vi "VCU MODEL CAN0.vi"() -> ()   [LabVIEW 2015]
uses:
  <vilib>/FPGAPlugInAG/cRIO-9063/niLvFpga_Open_cRIO-9063.vi
  <vilib>/rvi/interface/common/dynamic/niFpgaDynamicAddResources.vi
  <vilib>/Utility/error.llb/Error Cluster From Error Code.vi
  <vilib>/rvi/errors/niLvFpgaAdjustHostInterfaceError.vi
  <vilib>/FPGAPlugInAG/Dynamic/niLvFpga_Close_Dynamic.vi
  <vilib>/rvi/interface/nirviOpenFPGA/nirviOpenFPGA.xnode
  FPGA Bitfiles/VCU-VEHICLEMODEL_FPGATarget_CANBasic(FPGA)_WVt1gIpoBPw.lvbitx
  Basic (FPGA) CAN Engine .vi
  <vilib>/rvi/interface/nirviReadWriteControl/nirviReadWriteControl.xnode
  <vilib>/rvi/interface/nirviCloseFPGA/nirviCloseFPGA.xnode
  <vilib>/rvi/interface/Simulation/niFpgaSimulationCallBeginRW.vi
  NiFpgaLv.dll
panel:
  in  "Route_leg":u16
  in  "Start":bool
  out "P":cluster{sgl, sgl}(graph)
  out "V":cluster{"Vx_PV":sgl, "Vy_PV":sgl}(graph)
  out "Loop time":sgl
  out "Old Timestamp":u64
  out "Timestamp":u64
  out "Delta_Px":sgl
  out "Delta_Vx":sgl
  out "Delta_Py":sgl
  out "Delta_Vy":sgl
  out "F_C (magnitude)":sgl
  out "Theta_C (direction)":sgl
  out "Vx_SP":sgl
  out "x_MV (SGL)":sgl
  out "x_MV+ (plus m_epsilon)":sgl
  out "y_MV (SGL)":sgl
  out "Vy_SP":sgl
  out "Inverse Tangent (SGL)":sgl
  in  "Px_SP":sgl
  in  "Py_SP":sgl
  out "Vy_PV":sgl
  out "Px_PV":sgl
  out "Py_PV":sgl
  out "Vx_PV":sgl
  out "No# Frames Received":i32
  out "No# Frames Sent":i32
  out "error out":errorcluster
  # "Output"
  # "Set Point"
  # "Sensor Values"
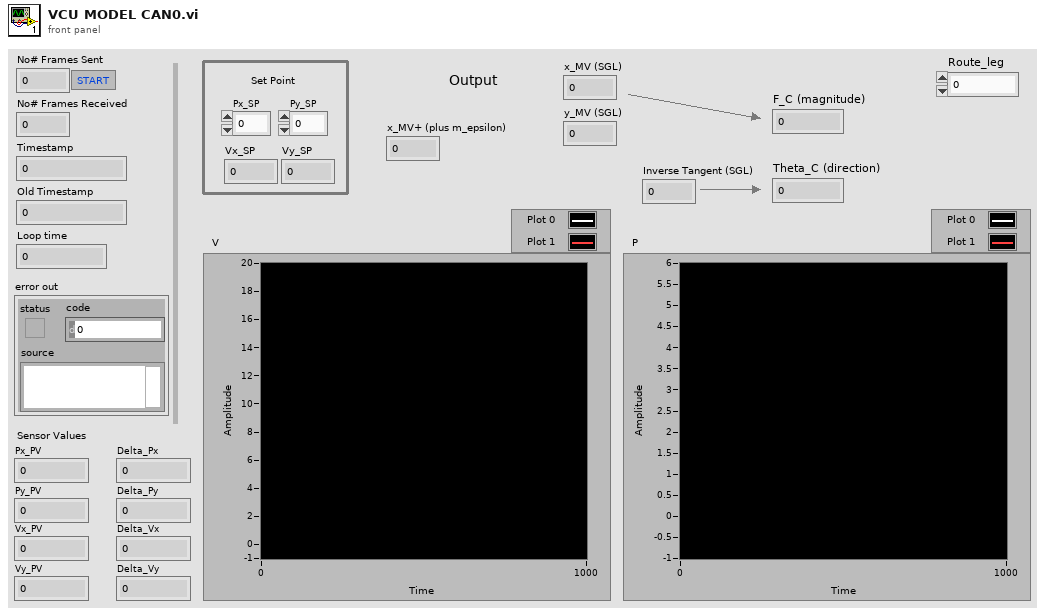
[diagram p1: front panel]
types:
  T1 = enum8{"Data Frame", "Remote Frame", "(reserved)", "(reserved) ", "(reserved)  ", "(reserved)   ", "Bus Error", "Transceiver Fault"}
  T2 = cluster{"timestamp high":u32, "timestamp low":u32, "identifier":u32, "type":enum8{"Data Frame", "Remote Frame", "(reserved)", "(reserved) ", "(reserved)  ", "(reserved)   ", "Bus Error", "Transceiver Fault"}, "info A":u8, "info B":u8, "data length":u8, "data":u8[]}
  T3 = cluster{u32, u32, u32, "type":enum8{"Data Frame", "Remote Frame", "(reserved)", "(reserved) ", "(reserved)  ", "(reserved)   ", "Bus Error", "Transceiver Fault"}, u8, u8, u8, u8[]}
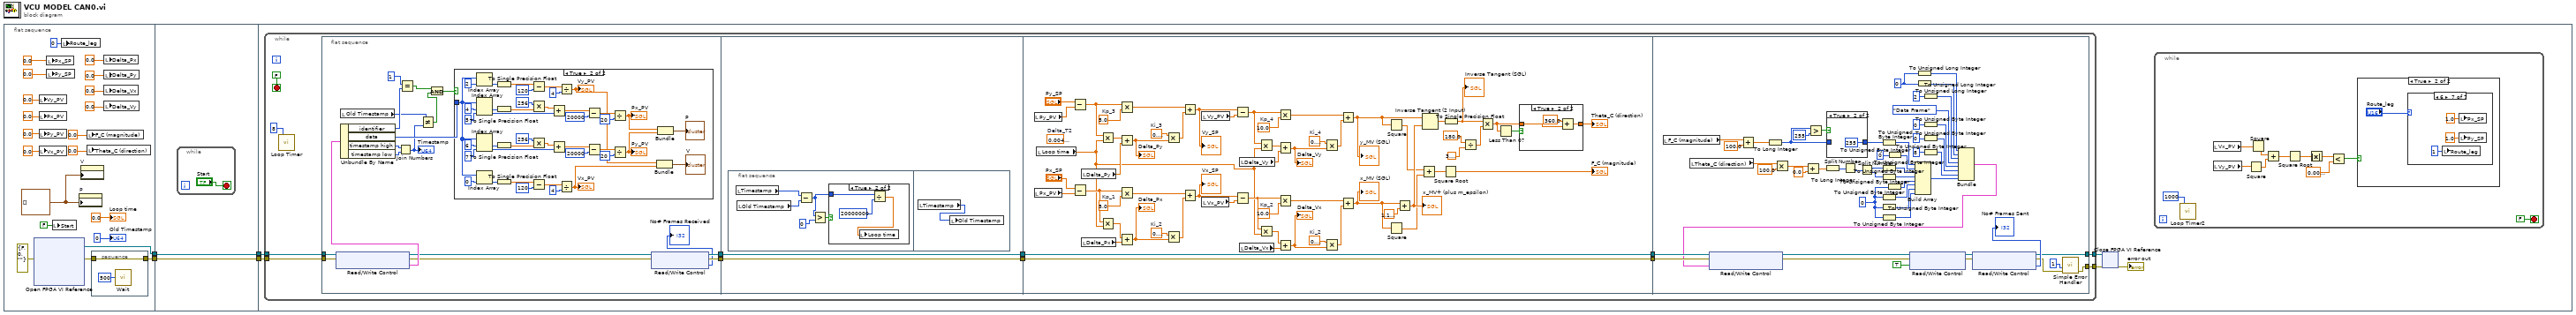
[diagram p0: block diagram]
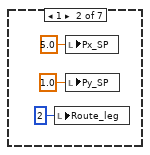
[diagram p4: hidden frame]
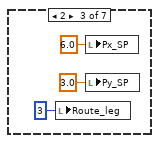
[diagram p5: hidden frame]
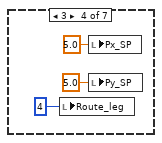
[diagram p6: hidden frame]
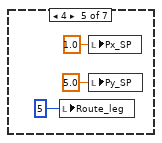
[diagram p7: hidden frame]
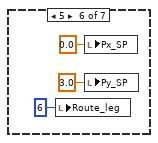
[diagram p8: hidden frame]
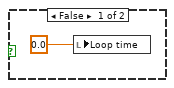
[diagram p10: hidden frame]
diagram:
  n1 = flat-sequence {
    tunnel: [w11] -> w4
    tunnel: [w10] -> w2
    tunnel: w4 -> [w29]
    tunnel: [w29] -> w3
    tunnel: w2 -> [w28]
    tunnel: [w28] -> w1
    tunnel: w3 -> [w32]
    tunnel: w1 -> [w31]
    frame #0 {
      w7 = cluster{"Px_PV":sgl, "Py_PV":sgl}[] [] ("History Data")
      n2 = xnode "Open FPGA VI Reference"("error in"=errorcluster {"status"=FALSE, "code"=0, "source"=""}) -> ("FPGA VI Reference Out"=w10:refnum<k20>, "error out"=w12:errorcluster)  [unwired: 1 in]
      n3 = local write "Vy_PV"(sgl 0.0 ("Vx_C")) -> ()
      n4 = local write "Px_PV"(sgl 0.0 ("Vy_C")) -> ()
      n5 = local write "Py_PV"(sgl 0.0 ("Px_C")) -> ()
      n6 = local write "Vx_PV"(sgl 0.0 ("Py_C")) -> ()
      n7 = local write "Px_SP"(sgl 0.0 ("Vx_C")) -> ()
      n8 = local write "Py_SP"(sgl 0.0 ("Vx_C")) -> ()
      n9 = local write "Start"(FALSE ("Start")) -> ()
      n10 = local write "Route_leg"(u16 0 ("Route_leg")) -> ()
      n11 = property on="P" class="WFChart (strict)"("History Data"=w7) -> ()  [unwired: 2 in, 2 out]
      n12 = property on="V" class="WFChart (strict)"("History Data"=w7) -> ()  [unwired: 2 in, 2 out]
      n13 = local write "F_C (magnitude)"(sgl 0.0 ("F_C")) -> ()
      n14 = local write "Theta_C (direction)"(sgl 0.0 ("Theta_C")) -> ()
      n15 = stacked-sequence {
        tunnel: w12 -> [w27]
        tunnel: [w27] -> w11
        frame #0 {
          n16 = call "Wait"("Count(mSec)"=u32 500) -> ()  [unwired: 1 out]
        }
      }
      n17 = local write "Delta_Px"(sgl 0.0 ("Delta_Px")) -> ()
      n18 = local write "Delta_Py"(sgl 0.0 ("Delta_Py")) -> ()
      n19 = local write "Delta_Vx"(sgl 0.0 ("Delta_Vx")) -> ()
      n20 = local write "Delta_Vy"(sgl 0.0) -> ()
      "Loop time" <- sgl 0.0 ("Loop time")
      "Old Timestamp" <- u64 0 ("Old Timestamp")
    }
    frame #1 {
      n21 = while {
        stop <- "Start" stop-if-true
      }
    }
    frame #2 {
      n22 = while {
        tunnel: [w76] -> w34
        tunnel: [w75] -> w33
        tunnel: w31 -> [w67]
        tunnel: w32 -> [w66]
        stop <- FALSE stop-if-true
        n23 = call "Loop Timer"("Count(mSec)"=u32 8) -> ()  [unwired: 1 out]
        n24 = flat-sequence {
          tunnel: [w91] -> w74
          tunnel: [w90] -> w72
          tunnel: w67 -> [w84]
          tunnel: w66 -> [w83]
          tunnel: w74 -> [w138]
          tunnel: [w138] -> w73
          tunnel: w72 -> [w137]
          tunnel: [w137] -> w71
          tunnel: w73 -> [w157]
          tunnel: w71 -> [w156]
          tunnel: [w157] -> w69
          tunnel: [w156] -> w68
          tunnel: [w214] -> w76
          tunnel: [w216] -> w75
          tunnel: w69 -> [w218]
          tunnel: w68 -> [w213]
          frame #0 {
            n25 = xnode "Read/Write Control"("FPGA VI Reference In"=w84, "error in"=w83) -> ("FPGA VI Reference Out"=w89:refnum<k20>, "error out"=w88:errorcluster, "CAN0 - Received Frame"=w94:T2)
            n26 = Unbundle By Name(w94) -> ("identifier"=w92:u32, "data"=w93:u8[], "timestamp high"=w86:u32, "timestamp low"=w85:u32)
            n27 = local read "Old Timestamp"() -> (w82:u64)
            n28 = Join Numbers(hi=w86, lo=w85) -> ((hi.lo)=w81:u64)
            "Timestamp" <- w81
            n29 = Equal?(x=u32 1, y=w92) -> (x = y?=w78:bool)
            n30 = Not Equal?(x=w82, y=w81) -> (x != y?=w79:bool)
            n31 = And(x=w78, y=w79) -> (x .and. y?=w80:bool)
            n32 = case shown="True" w80 {
              tunnel: w93 -> [_ w102]
              frame False {
              }
              frame True {
                n33 = Index Array(array=w102, index=2 ("索引")) -> (element=w110:u8)
                n34 = Index Array(array=w102, index #1=4 ("索引"), index #2=5 ("索引")) -> (element #1=w108:u8, element #2=w103:u8)
                n35 = Index Array(array=w102, index #1=6 ("索引"), index #2=7 ("索引")) -> (element #1=w106:u8, element #2=w122:u8)
                n36 = Index Array(array=w102, index=0 ("索引")) -> (element=w111:u8)
                n37 = To Single Precision Float(number=w110) -> (single precision float=w109:sgl)
                n38 = To Single Precision Float(number=w108) -> (single precision float=w107:sgl)
                n39 = To Single Precision Float(number=w106) -> (single precision float=w105:sgl)
                n40 = To Single Precision Float(number=w111) -> (single precision float=w112:sgl)
                n41 = Subtract(x=w109, y=u32 120) -> (x-y=w115:sgl)
                n42 = Multiply(x=u32 256 ("y"), y=w107) -> (x*y=w130:sgl)
                n43 = Multiply(x=u32 256 ("y"), y=w105) -> (x*y=w123:sgl)
                n44 = Subtract(x=w112, y=u32 120) -> (x-y=w135:sgl)
                n45 = Add(x=w130, y=w103) -> (x+y=w128:sgl)
                n46 = Add(x=w123, y=w122) -> (x+y=w120:sgl)
                n47 = Divide(x=w115, y=u32 4) -> (x/y=w97:sgl)
                "Vy_PV" <- w97
                n48 = Divide(x=w135, y=u32 4) -> (x/y=w96:sgl)
                "Vx_PV" <- w96
                n49 = Subtract(x=w128, y=u32 20000) -> (x-y=w126:sgl)
                n50 = Subtract(x=w120, y=u32 20000) -> (x-y=w118:sgl)
                n51 = Divide(x=w126, y=u32 20) -> (x/y=w101:sgl)
                "Px_PV" <- w101
                n52 = Divide(x=w118, y=u32 20) -> (x/y=w100:sgl)
                "Py_PV" <- w100
                n53 = Bundle(w97, w96) -> (→"V":cluster{sgl, sgl})  [unwired: 1 in]
                n54 = Bundle(w101, w100) -> (→"P":cluster{sgl, sgl})  [unwired: 1 in]
              }
            }
            n55 = xnode "Read/Write Control"("FPGA VI Reference In"=w89, "error in"=w88) -> ("FPGA VI Reference Out"=w91:refnum<k20>, "error out"=w90:errorcluster, "CAN0 -  Received"=→"No# Frames Received":u32)
          }
          frame #1 {
            n56 = flat-sequence {
              frame #0 {
                n57 = local read "Timestamp"() -> (w142:u64)
                n58 = local read "Old Timestamp"() -> (w143:u64)
                n59 = Subtract(x=w142, y=w143) -> (x-y=w140:u64)
                n60 = Greater?(x=w140, y=u64 0) -> (0:w141:bool)
                n61 = case shown="True" w141 {
                  tunnel: w140 -> [_ w147]
                  frame False {
                    n62 = local write "Loop time"(sgl 0.0 ("Loop time")) -> ()
                  }
                  frame True {
                    n63 = Divide(x=w147, y=u64 20000000) -> (x/y=w145:dbl)
                    n64 = local write "Loop time"(w145) -> ()
                  }
                }
              }
              frame #1 {
                n65 = local read "Timestamp"() -> (w148:u64)
                n66 = local write "Old Timestamp"(w148) -> ()
              }
            }
          }
          frame #2 {
            w201 = sgl 0.1  # Ki_2
            w166 = sgl 0.1  # Ki_2
            w197 = sgl 0.1  # Ki_4
            w194 = sgl 0.1  # Ki_3
            w182 = sgl 10.0  # Kp_4
            w179 = sgl 5.0  # Kp_3
            w173 = sgl 10.0  # Kp_2
            (unwired) sgl 0.005  # Delta_T2
            w169 = sgl 5.0  # Kp_1
            n67 = local read "Py_PV"() -> (w186:sgl)
            n68 = local read "Px_PV"() -> (w168:sgl)
            n69 = local read "Loop time"() -> (w155:sgl)
            n70 = Subtract(x="Py_SP", y=w186) -> (x-y=w180:sgl)
            n71 = Subtract(x="Px_SP", y=w168) -> (x-y=w164:sgl)
            n72 = local read "Delta_Py"() -> (w189:sgl)
            n73 = local read "Delta_Px"() -> (w172:sgl)
            n74 = Multiply(x=w180, y=w155) -> (x*y=w188:sgl)
            n75 = Multiply(x=w164, y=w155) -> (x*y=w171:sgl)
            n76 = Multiply(x=w180, y=w179) -> (x*y=w181:sgl)
            n77 = Add(x=w188, y=w189) -> (x+y=w195:sgl)
            "Delta_Py" <- w195
            n78 = Multiply(x=w164, y=w169) -> (x*y=w170:sgl)
            n79 = Add(x=w171, y=w172) -> (x+y=w203:sgl)
            "Delta_Px" <- w203
            n80 = Multiply(x=w194, y=w195) -> (x*y=w196:sgl)
            n81 = Multiply(x=w201, y=w203) -> (x*y=w202:sgl)
            n82 = Add(x=w181, y=w196) -> (x+y=w184:sgl)
            "Vy_SP" <- w184
            n83 = Add(x=w170, y=w202) -> (x+y=w175:sgl)
            "Vx_SP" <- w175
            n84 = local read "Vy_PV"() -> (w187:sgl)
            n85 = local read "Vx_PV"() -> (w176:sgl)
            n86 = Subtract(x=w184, y=w187) -> (x-y=w183:sgl)
            n87 = Subtract(x=w175, y=w176) -> (x-y=w174:sgl)
            n88 = local read "Delta_Vy"() -> (w190:sgl)
            n89 = local read "Delta_Vx"() -> (w178:sgl)
            n90 = Multiply(x=w183, y=w155) -> (x*y=w185:sgl)
            n91 = Multiply(x=w174, y=w155) -> (x*y=w177:sgl)
            n92 = Multiply(x=w183, y=w182) -> (x*y=w191:sgl)
            n93 = Add(x=w185, y=w190) -> (x+y=w198:sgl)
            "Delta_Vy" <- w198
            n94 = Multiply(x=w174, y=w173) -> (x*y=w163:sgl)
            n95 = Add(x=w177, y=w178) -> (x+y=w165:sgl)
            "Delta_Vx" <- w165
            n96 = Multiply(x=w197, y=w198) -> (x*y=w199:sgl)
            n97 = Multiply(x=w166, y=w165) -> (x*y=w200:sgl)
            n98 = Add(x=w191, y=w199) -> (x+y=w160:sgl)
            "y_MV (SGL)" <- w160
            n99 = Add(x=w163, y=w200) -> (x+y=w204:sgl)
            "x_MV (SGL)" <- w204
            n100 = Square(x=w160) -> (x^2=w153:sgl)
            n101 = Square(x=w204) -> (x^2=w154:sgl)
            n102 = Add(x=w204, y=sgl 1.1920929e-07) -> (x+y=w158:sgl)
            "x_MV+ (plus m_epsilon)" <- w158
            n103 = Add(x=w153, y=w154) -> (x+y=w192:sgl)
            n104 = Inverse Tangent (2 Input)(1:w158, 2:w160) -> (0:w159:sgl)
            n105 = Square Root(x=w192) -> (sqrt(x)=→"F_C (magnitude)":sgl)
            n106 = To Single Precision Float(number=w159) -> (single precision float=w167:sgl)
            "Inverse Tangent (SGL)" <- w167
            n107 = Divide(x=sgl 180.0 ("y"), y=sgl 3.1415927) -> (x/y=w149:sgl)
            n108 = Multiply(x=w167, y=w149) -> (x*y=w206:sgl)
            n109 = Less Than 0?(x=w206) -> (x < 0?=w205:bool)
            n110 = case shown="True" w205 {
              tunnel: w206 -> [w208 w211]
              tunnel: [w208 w209] -> w207
              frame False {
              }
              frame True {
                n111 = Add(x=sgl 360.0, y=w211) -> (x+y=w209:sgl)
              }
            }
            "Theta_C (direction)" <- w207
          }
          frame #3 {
            w225 = i16 0
            w256 = i16 0
            n112 = local read "F_C (magnitude)"() -> (w263:sgl)
            n113 = local read "Theta_C (direction)"() -> (w235:sgl)
            n114 = Add(x=w263, y=sgl 100.0) -> (x+y=w259:sgl)
            n115 = To Long Integer(number=w259) -> (32bit integer=w262:i32)
            n116 = Multiply(x=w235, y=sgl 100.0) -> (x*y=w232:sgl)
            n117 = Add(x=w232, y=sgl 0.0) -> (x+y=w234:sgl)
            n118 = Greater?(x=w262, y=255) -> (0:w260:bool)
            n119 = To Long Integer(number=w234) -> (32bit integer=w230:i32)
            n120 = case shown="True" w260 {
              tunnel: w262 -> [w264 _]
              tunnel: [w264 255] -> w236
              frame False {
              }
              frame True {
              }
            }
            n121 = Split Number(x=w230) -> (lo(x)=w229:u16)  [unwired: 1 out]
            n122 = Split Number(x=w229) -> (hi(x)=w228:u8, lo(x)=w227:u8)
            n123 = To Unsigned Byte Integer(number=w236) -> (unsigned 8bit integer=w246:u8)
            n124 = To Unsigned Byte Integer(number=w228) -> (unsigned 8bit integer=w244:u8)
            n125 = To Unsigned Byte Integer(number=w227) -> (unsigned 8bit integer=w243:u8)
            n126 = To Unsigned Byte Integer(number=w225) -> (unsigned 8bit integer=w241:u8)
            n127 = To Unsigned Byte Integer(number=w225) -> (unsigned 8bit integer=w240:u8)
            n128 = To Unsigned Byte Integer(number=w225) -> (unsigned 8bit integer=w239:u8)
            n129 = To Unsigned Byte Integer(number=w225) -> (unsigned 8bit integer=w242:u8)
            n130 = To Unsigned Byte Integer(number=i16 0) -> (unsigned 8bit integer=w245:u8)
            n131 = Build Array(w246, w245, w244, w243, w242, w241, w240, w239) -> (w237:u8[])
            n132 = To Unsigned Long Integer(number=w256) -> (unsigned 32bit integer=w252:u32)
            n133 = To Unsigned Long Integer(number=w256) -> (unsigned 32bit integer=w251:u32)
            n134 = To Unsigned Long Integer(number=i16 2) -> (unsigned 32bit integer=w250:u32)
            n135 = To Unsigned Byte Integer(number=u8 0 ("info A")) -> (unsigned 8bit integer=w249:u8)
            n136 = To Unsigned Byte Integer(number=u8 0 ("info B")) -> (unsigned 8bit integer=w248:u8)
            n137 = To Unsigned Byte Integer(number=i16 8) -> (unsigned 8bit integer=w247:u8)
            n138 = Bundle(w252, w251, w250, "type"=T1."Data Frame", w249, w248, w247, w237) -> (w212:T3)  [unwired: 1 in]
            n139 = xnode "Read/Write Control"("FPGA VI Reference In"=w218, "error in"=w213, "CAN0 - Transmit Frame"=w212) -> ("FPGA VI Reference Out"=w217:refnum<k20>, "error out"=w215:errorcluster)
            n140 = xnode "Read/Write Control"("FPGA VI Reference In"=w217, "error in"=w215, "CAN0 - Transmit"=TRUE) -> ("FPGA VI Reference Out"=w221:refnum<k20>, "error out"=w224:errorcluster)
            n141 = xnode "Read/Write Control"("FPGA VI Reference In"=w221, "error in"=w224) -> ("FPGA VI Reference Out"=w216:refnum<k20>, "error out"=w222:errorcluster, "CAN0 - Frames Sent"=→"No# Frames Sent":u32)
            n142 = call <vilib>:"Simple Error Handler.vi"("type of dialog (OK msg:1)"=1, "error in (no error)"=w222) -> ("error out"=w214:errorcluster)  [unwired: 3 in, 4 out]
          }
        }
      }
      n143 = xnode "Close FPGA VI Reference"("FPGA VI Reference In"=w33, "error in"=w34) -> ("error out"=→"error out":errorcluster)
      n144 = while {
        stop <- FALSE stop-if-true
        n145 = call "Loop Timer2"("Count(mSec)"=u32 1000) -> ()  [unwired: 1 out]
        n146 = local read "Vx_PV"() -> (w37:sgl)
        n147 = local read "Vy_PV"() -> (w38:sgl)
        n148 = Square(x=w38) -> (x^2=w41:sgl)
        n149 = Square(x=w37) -> (x^2=w40:sgl)
        n150 = Add(x=w40, y=w41) -> (x+y=w39:sgl)
        n151 = Square Root(x=w39) -> (sqrt(x)=w44:sgl)
        n152 = Absolute Value(x=w44) -> (abs(x)=w43:sgl)
        n153 = Less?(x=w43, y=sgl 0.01) -> (x < y?=w45:bool)
        n154 = case shown="True" w45 {
          frame False {
          }
          frame True {
            n155 = case shown="6" "Route_leg" {
              frame Default {
              }
              frame 1 {
                n156 = local write "Route_leg"(u16 2 ("Route_leg")) -> ()
                n157 = local write "Px_SP"(sgl 5.0 ("Px_SP")) -> ()
                n158 = local write "Py_SP"(sgl 1.0 ("Py_SP")) -> ()
              }
              frame 2 {
                n159 = local write "Route_leg"(u16 3 ("Route_leg")) -> ()
                n160 = local write "Px_SP"(sgl 6.0 ("Px_SP")) -> ()
                n161 = local write "Py_SP"(sgl 3.0 ("Py_SP")) -> ()
              }
              frame 3 {
                n162 = local write "Route_leg"(u16 4 ("Route_leg 2")) -> ()
                n163 = local write "Px_SP"(sgl 5.0 ("Px_SP")) -> ()
                n164 = local write "Py_SP"(sgl 5.0 ("Py_SP")) -> ()
              }
              frame 4 {
                n165 = local write "Route_leg"(u16 5 ("Route_leg 2")) -> ()
                n166 = local write "Px_SP"(sgl 1.0 ("Px_SP")) -> ()
                n167 = local write "Py_SP"(sgl 5.0 ("Py_SP")) -> ()
              }
              frame 5 {
                n168 = local write "Route_leg"(u16 6 ("Route_leg")) -> ()
                n169 = local write "Px_SP"(sgl 0.0 ("Px_SP")) -> ()
                n170 = local write "Py_SP"(sgl 3.0 ("Py_SP")) -> ()
              }
              frame 6 {
                n171 = local write "Route_leg"(u16 1 ("Route_leg")) -> ()
                n172 = local write "Px_SP"(sgl 1.0 ("Px_SP")) -> ()
                n173 = local write "Py_SP"(sgl 1.0 ("Py_SP")) -> ()
              }
            }
          }
        }
      }
    }
  }
